vi "Add Subsystem Dialog.vi"(8 "error in (no error)":errorcluster, 11 "Existing Subsystems":string[](array[string])) -> (0 "error out":errorcluster, 1 "OK?":bool caption="OK", 2 "URL Out":string caption="URL", 3 "Subsystem Name Out":string caption="Subsystem Name")   [LabVIEW 2024]
doc: "This VI is a user interface VI and is used to add a subsystem."
panel:
  in  "OK":bool
  out "Subsystem URL Not Modified?":bool
  out "Subsystem Name Not Modified?":bool
  in  "URL":string="Example: \\\\localhost\\cRIO\\Subsystem IO Template"
  in  "Subsystem Name":string="Subsystem"
  in  "Cancel":bool
  # "Note: \nURL specifies the URL of the real device which you want to bind the subsystem to. The URL must exist in the engine."
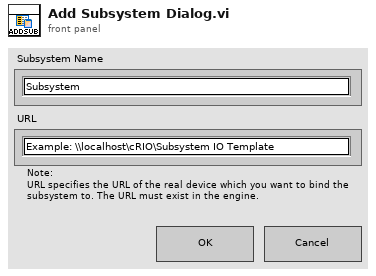
[diagram p1: front panel]
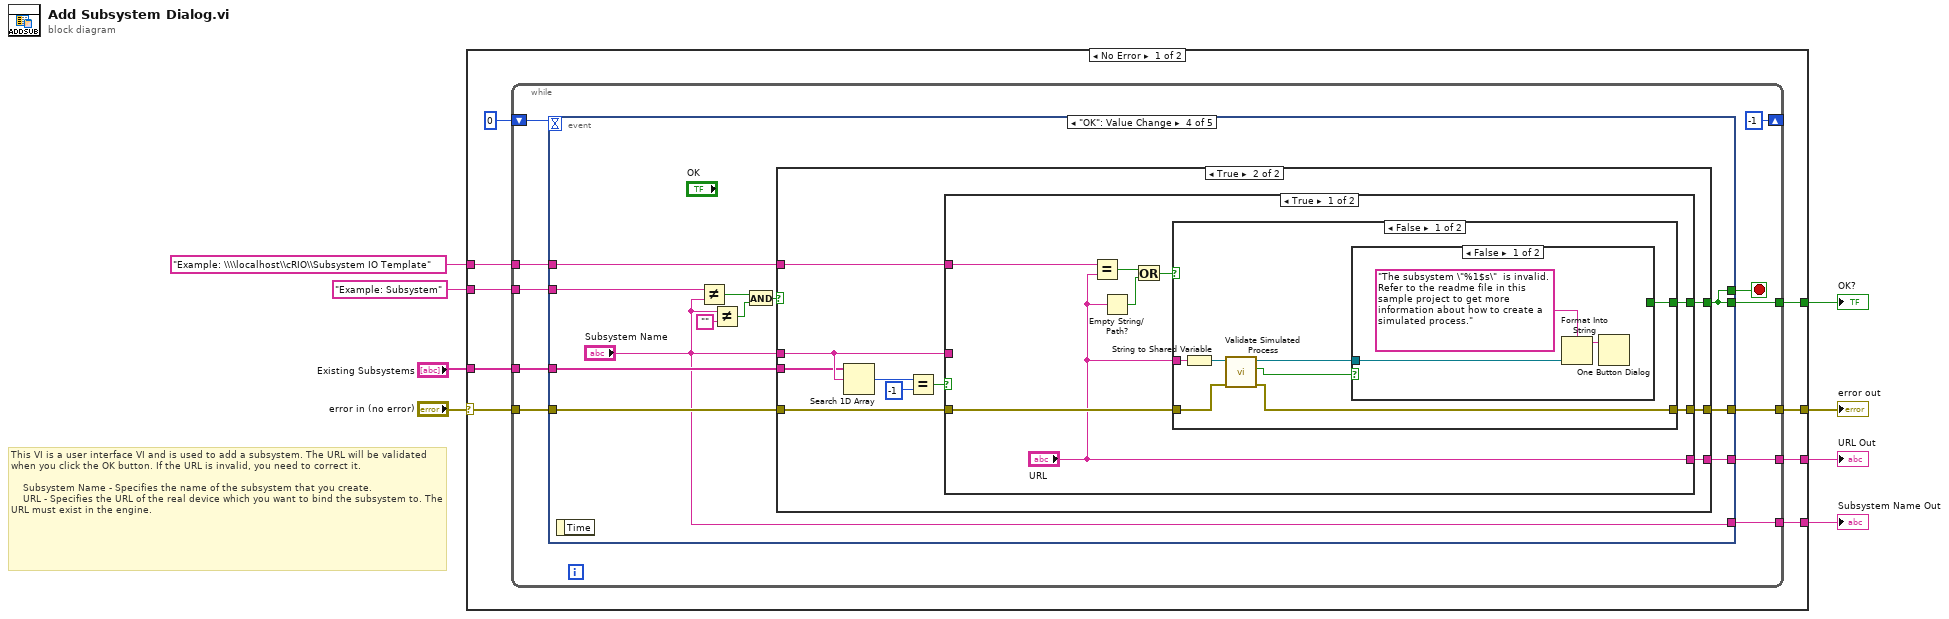
[diagram p0: block diagram]
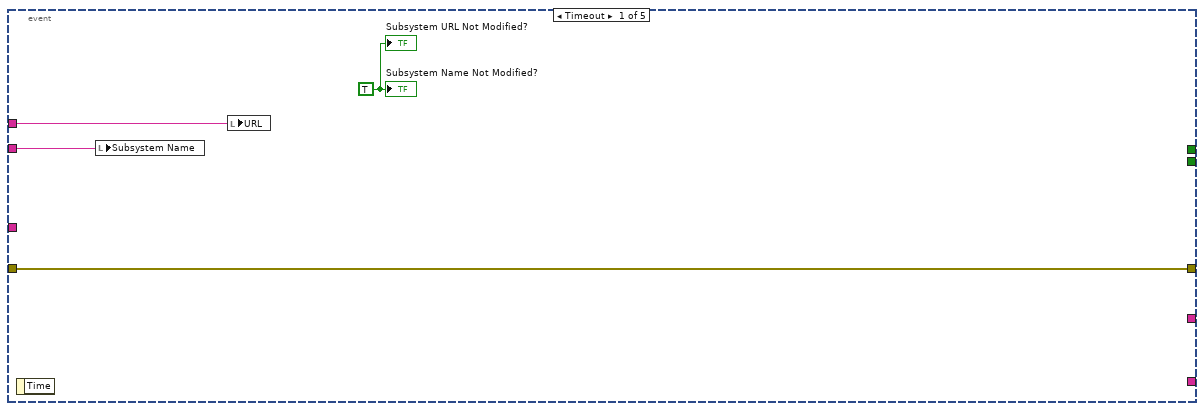
[diagram p2: hidden frame]
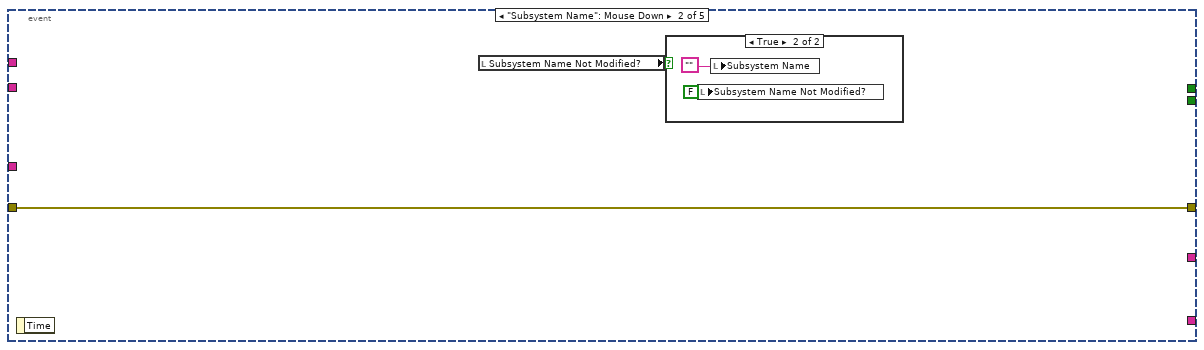
[diagram p3: hidden frame]
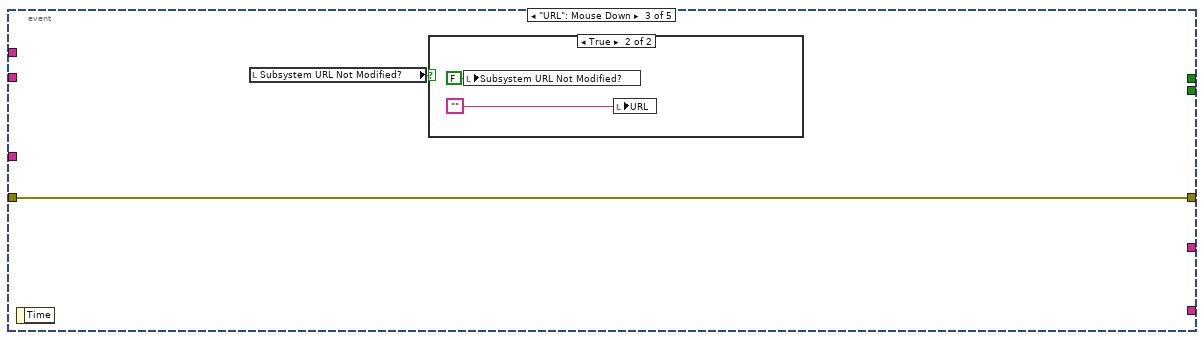
[diagram p5: hidden frame]
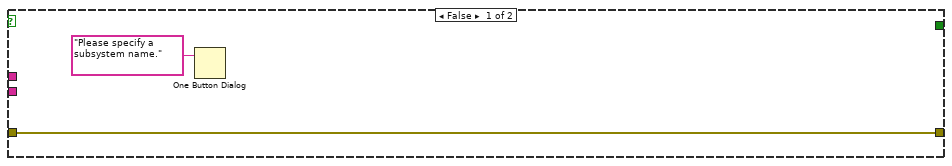
[diagram p7: hidden frame]
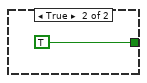
[diagram p8: hidden frame]
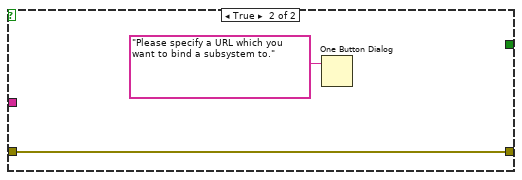
[diagram p9: hidden frame]
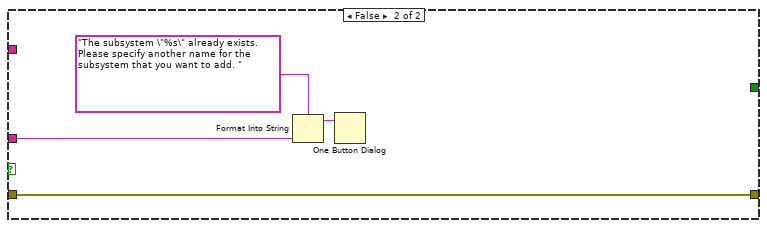
[diagram p10: hidden frame]
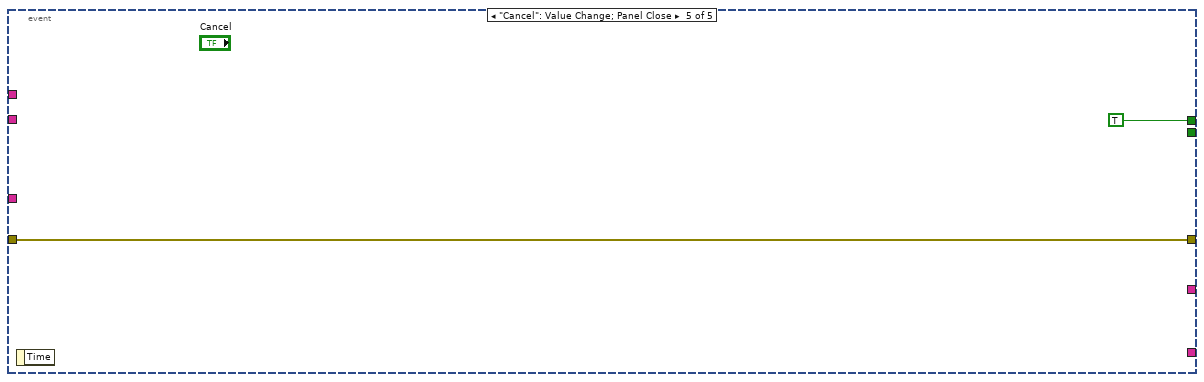
[diagram p11: hidden frame]
diagram:
  # "This VI is a user interface VI and is used to add a subsystem. The URL will be validated when you click the OK button. If the URL is invalid, you need to correct it.\n\n    Subsystem Name - Specifies the name of the subsystem that you create. \n    URL - Specifies the URL of the real device which you want to bind the subsystem to. The URL must exist in the engine."
  n1 = case shown="No Error" "error in (no error)" {
    selector: "error in (no error)" -> [w9 w92]
    tunnel: [w12 w92] -> w8
    tunnel: [w17 _] -> w7
    tunnel: "Example: \\\\localhost\\cRIO\\Subsystem IO Template" ("URL") -> [w15 _]
    tunnel: "Example: Subsystem" ("Subsystem Name") -> [w14 _]
    tunnel: "Existing Subsystems" -> [w13 _]
    tunnel: [w11 _] -> w2
    tunnel: [w10 _] -> w1
    frame No Error {
      n2 = while {
        tunnel: [w27] -> w17
        shift-right: [-1] -> _
        shift-left: 0 -> [w26]
        tunnel: w15 -> [w25]
        tunnel: w14 -> [w24]
        tunnel: w13 -> [w22]
        tunnel: [w21] -> w12
        tunnel: [w20] -> w11
        tunnel: [w19] -> w10
        tunnel: w9 -> [w18]
        stop <- w28 stop-if-true
        n3 = event shown="[3] \"OK\": Value Change" {
          selector: _ -> [_ _ _ _ _]
          dyn-events: _ -> [_ _ _ _ _]
          timeout: w26 -> [_ _ _ _ _]
          tunnel: [_ _ _ w46 TRUE] -> w28
          tunnel: [_ _ _ w46 _] -> w27
          tunnel: w25 -> [w31 _ _ w47 _]
          tunnel: w24 -> [w30 _ _ w52 _]
          tunnel: w22 -> [_ _ _ w45 _]
          tunnel: [w29 w33 w37 w44 w90] -> w21
          tunnel: [_ _ _ "Subsystem Name" _] -> w20
          tunnel: [_ _ _ w43 _] -> w19
          tunnel: w18 -> [w29 w33 w37 w42 w90]
          event Timeout {
            w32 = TRUE ("Subsystem URL 1st time?")
            n4 = event-data() -> ()  [unwired: 1 in, 1 out]
            n5 = local write "Subsystem Name"(w30) -> ()
            n6 = local write "URL"(w31) -> ()
            "Subsystem Name Not Modified?" <- w32
            "Subsystem URL Not Modified?" <- w32
          }
          event "Subsystem Name": Mouse Down {
            n7 = event-data() -> ()  [unwired: 1 in, 1 out]
            n8 = local read "Subsystem Name Not Modified?"() -> (w34:bool)
            n9 = case shown="True" w34 {
              frame False {
              }
              frame True {
                n10 = local write "Subsystem Name Not Modified?"(FALSE ("Subsystem URL 1st time?")) -> ()
                n11 = local write "Subsystem Name"("" ("Subsystem Name")) -> ()
              }
            }
          }
          event "URL": Mouse Down {
            n12 = event-data() -> ()  [unwired: 1 in, 1 out]
            n13 = local read "Subsystem URL Not Modified?"() -> (w38:bool)
            n14 = case shown="True" w38 {
              frame False {
              }
              frame True {
                n15 = local write "Subsystem URL Not Modified?"(FALSE ("Subsystem URL 1st time?")) -> ()
                n16 = local write "URL"("" ("Subsystem Name")) -> ()
              }
            }
          }
          event "OK": Value Change {
            n17 = event-data() -> ()  [unwired: 1 in, 1 out]
            n18 = Not Equal?(x=w52, y="Subsystem Name") -> (x != y?=w50:bool)
            n19 = Not Equal?(x="Subsystem Name", y="") -> (x != y?=w49:bool)
            n20 = And(x=w50, y=w49) -> (x .and. y?=w48:bool)
            n21 = case shown="True" w48 {
              tunnel: "Subsystem Name" -> [_ w63]
              tunnel: w47 -> [_ w60]
              tunnel: [_ w59] -> w46
              tunnel: w45 -> [_ w58]
              tunnel: [w53 w57] -> w44
              tunnel: [_ w56] -> w43
              tunnel: w42 -> [w53 w55]
              frame False {
                n22 = One Button Dialog(message="Please specify a subsystem name.") -> ()  [unwired: 1 in, 1 out]
              }
              frame True {
                n23 = Search 1D Array(1D array=w58, element=w63) -> (index of element=w64:i32)  [unwired: 1 in]
                n24 = Equal?(x=w64, y=-1) -> (x = y?=w61:bool)
                n25 = case shown="True" w61 {
                  tunnel: w63 -> [_ w89]
                  tunnel: w60 -> [w70 _]
                  tunnel: [w69 _] -> w59
                  tunnel: [w67 w86] -> w57
                  tunnel: ["URL" _] -> w56
                  tunnel: w55 -> [w66 w86]
                  frame True {
                    n26 = Equal?(x=w70, y="URL") -> (x = y?=w72:bool)
                    n27 = Empty String/Path?(string/path="URL") -> (empty?=w68:bool)
                    n28 = Or(x=w72, y=w68) -> (x .or. y?=w71:bool)
                    n29 = case shown="False" w71 {
                      tunnel: "URL" -> [w79 _]
                      tunnel: [w78 _] -> w69
                      tunnel: [w74 w84] -> w67
                      tunnel: w66 -> [w73 w84]
                      frame False {
                        n30 = String to Shared Variable(0:w79) -> (2:w77:refnum<k21>)  [unwired: 1 out]
                        n31 = call "Validate Simulated Process.vi"("error in (no error)"=w73, "URL"=w77) -> ("error out"=w74:errorcluster, "Valid?"=w75:bool, "dup URL"=w76:refnum<k21>)  [unwired: 7 in]
                        n32 = case shown="False" w75 {
                          tunnel: w76 -> [w80 _]
                          tunnel: [_ TRUE] -> w78
                          frame False {
                            n33 = Format Into String(format string="The subsystem \"%1$s\"  is invalid. Refer to the readme file in this sample project to get more information about how to create a simulated process." ("message"), w80) -> (resulting string=w81:string)  [unwired: 2 in, 1 out]
                            n34 = One Button Dialog(message=w81) -> ()  [unwired: 1 in, 1 out]
                          }
                          frame True {
                          }
                        }
                      }
                      frame True {
                        n35 = One Button Dialog(message="Please specify a URL which you want to bind a subsystem to.") -> ()  [unwired: 1 in, 1 out]
                      }
                    }
                  }
                  frame False {
                    n36 = Format Into String(format string="The subsystem \"%s\" already exists. Please specify another name for the subsystem that you want to add. " ("message"), w89) -> (resulting string=w88:string)  [unwired: 2 in, 1 out]
                    n37 = One Button Dialog(message=w88) -> ()  [unwired: 1 in, 1 out]
                  }
                }
              }
            }
          }
          event "Cancel": Value Change; Panel Close {
            n38 = event-data() -> ()  [unwired: 1 in, 1 out]
          }
        }
      }
    }
    frame Error {
    }
  }
  "error out" <- w8
  "OK?" <- w7
  "Subsystem Name Out" <- w2
  "URL Out" <- w1
